vi "Init and Rotate array Graf.vi"(5 "Reset":bool, 7 "Stop read":bool, 9 "Array size":i32=30, 10 "PV":dbl[](array[numeric]), 11 "XY Graf in":cluster{"time stamp":timestamp[], "PV":dbl[]}[](array[cluster])) -> (3 "XY Graf out":cluster{"time stamp":timestamp[], "PV":dbl[]}[](array[cluster]))   [LabVIEW 2019, in "Userlib.lvlib"]
uses:
  Userlib.lvlib
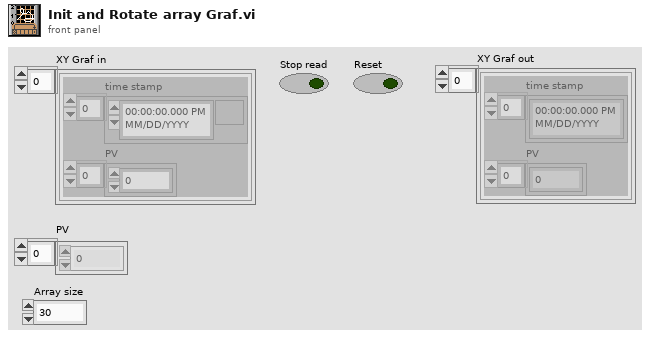
[diagram p1: front panel]
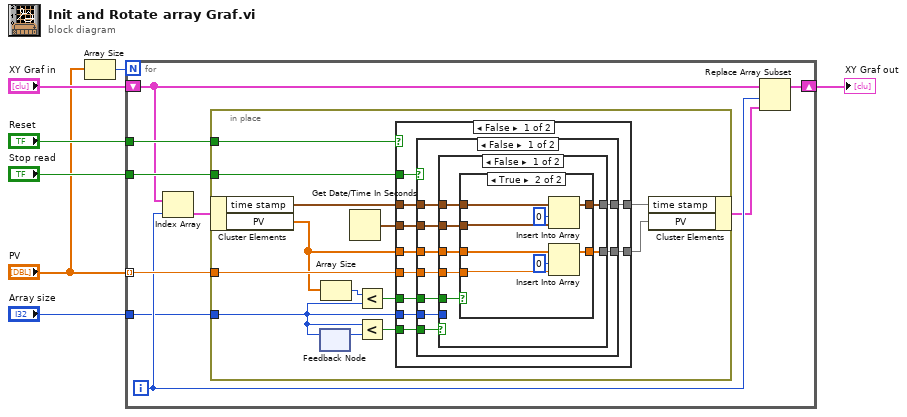
[diagram p0: block diagram]
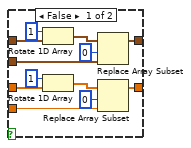
[diagram p2: hidden frame]
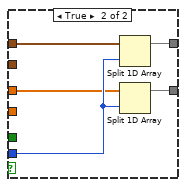
[diagram p3: hidden frame]
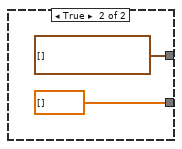
[diagram p5: hidden frame]
diagram:
  n1 = Array Size(array="PV") -> (size(s)=w2:i32)
  n2 = for {
    N: w2 -> [_]
    tunnel: "Stop read" -> [w16]
    tunnel: "Reset" -> [w15]
    tunnel: "PV" -> [w14] mode=indexing
    tunnel: "Array size" -> [w11]
    shift-right: [w10] -> w4
    shift-left: "XY Graf in" -> [w12]
    i -> [w13]
    n3 = Index Array(array=w12, index=w13) -> (element=w9:cluster{"time stamp":timestamp[], "PV":dbl[]})
    n4 = in-place {
      in-place-border: w16 -> [w29]
      in-place-border: w15 -> [w24]
      in-place-border: w14 -> [w27]
      in-place-border: w11 -> [w20]
      n5 = in-place-cluster #1(w9) -> ("time stamp"=w25:timestamp[], "PV"=w19:dbl[])
      n6 = feedback #2() -> (w23:i32)  [unwired: 1 in]
      n7 = feedback-in #2(w20) -> ()
      n8 = Array Size(array=w19) -> (size(s)=w28:i32)
      n9 = Get Date/Time In Seconds() -> (seconds since 1Jan1904=w26:timestamp)
      n10 = Less?(x=w28, y=w20) -> (x < y?=w18:bool)
      n11 = Less?(x=w20, y=w23) -> (x < y?=w22:bool)
      n12 = case shown="False" w24 {
        tunnel: w29 -> [w31 _]
        tunnel: w27 -> [w39 _]
        tunnel: w26 -> [w38 _]
        tunnel: [w37 timestamp[] [] ("time stamp")] -> w21
        tunnel: w25 -> [w36 _]
        tunnel: w19 -> [w35 _]
        tunnel: [w34 dbl[] [] ("PV")] -> w17
        tunnel: w22 -> [w30 _]
        tunnel: w20 -> [w33 _]
        tunnel: w18 -> [w32 _]
        frame False {
          n13 = case shown="False" w31 {
            tunnel: w30 -> [w42 _]
            tunnel: w39 -> [w48 _]
            tunnel: w38 -> [w47 _]
            tunnel: [w46 w82] -> w37
            tunnel: w36 -> [w45 w82]
            tunnel: w35 -> [w44 w81]
            tunnel: [w43 w81] -> w34
            tunnel: w33 -> [w40 _]
            tunnel: w32 -> [w41 _]
            frame False {
              n14 = case shown="False" w42 {
                tunnel: w48 -> [w55 _]
                tunnel: w47 -> [w54 _]
                tunnel: w45 -> [w53 w78]
                tunnel: w44 -> [w52 w79]
                tunnel: [w51 w76] -> w43
                tunnel: [w50 w77] -> w46
                tunnel: w41 -> [w49 _]
                tunnel: w40 -> [_ w80]
                frame False {
                  n15 = case shown="True" w49 {
                    tunnel: w53 -> [w64 w73]
                    tunnel: w54 -> [w63 w68]
                    tunnel: w52 -> [w59 w72]
                    tunnel: w55 -> [w58 w69]
                    tunnel: [w57 w71] -> w50
                    tunnel: [w56 w70] -> w51
                    frame False {
                      n16 = Rotate 1D Array(1:w64, 2:1 ("n")) -> (0:w66:timestamp[])
                      n17 = Rotate 1D Array(1:w59, 2:1 ("n")) -> (0:w61:dbl[])
                      n18 = Replace Array Subset(array=w66, new element=w63, index=0) -> (w57:timestamp[])
                      n19 = Replace Array Subset(array=w61, new element=w58, index=0) -> (w56:dbl[])
                    }
                    frame True {
                      n20 = Insert Into Array(array=w73, index=0, new element=w68) -> (w71:timestamp[])
                      n21 = Insert Into Array(array=w72, index=0, new element=w69) -> (w70:dbl[])
                    }
                  }
                }
                frame True {
                  n22 = Split 1D Array(array=w78, index=w80) -> (first subarray=w77:timestamp[])  [unwired: 1 out]
                  n23 = Split 1D Array(array=w79, index=w80) -> (first subarray=w76:dbl[])  [unwired: 1 out]
                }
              }
            }
            frame True {
            }
          }
        }
        frame True {
        }
      }
      n24 = in-place-cluster #1("time stamp"=w21, "PV"=w17) -> (w8:cluster{"time stamp":timestamp[], "PV":dbl[]})
    }
    n25 = Replace Array Subset(array=w12, new element=w8, index=w13) -> (w10:cluster{"time stamp":timestamp[], "PV":dbl[]}[])
  }
  "XY Graf out" <- w4
